vi "PCO_GetExpTrigSignalStatus.vi"(8 "error in (no error)":errorcluster {"code" format="%x"}, 11 "ph":u64) -> (0 "error out":errorcluster {"code" format="%x"}, 1 "wExpTrgSignal":u16(ring) items=["OFF", "ON"], 2 "ErrorMessage":i32 format="%x", 3 "ph out":u64)   [LabVIEW 2019, in "SDK.lvlib" / "TimingControl.lvlib"]
doc: "<b>Description:</b>\nThis function returns the current status of the <exp trig> input line.\nSee respective camera manual for more information about hardware signals.\n\nDue to response and processing times the delay between the software delivered status and the current status may be several milliseconds. For instance caused by interface and / or operating system.\n\n<b>Supported camera type:</b>\npco.pixelfly usb, pco.ultraviolet, pco.1300, pco.1400\n\n<b>Descriptor dependency:</b>\nNone"
uses:
  TimingControl.lvlib
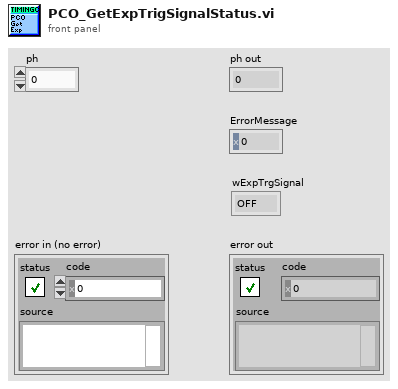
[diagram p1: front panel]
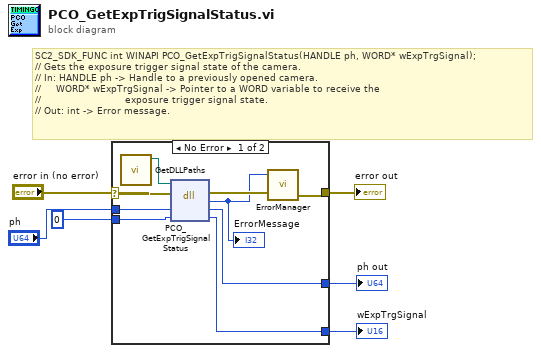
[diagram p0: block diagram]
diagram:
  # "SC2_SDK_FUNC int WINAPI PCO_GetExpTrigSignalStatus(HANDLE ph, WORD* wExpTrgSignal);\n// Gets the exposure trigger signal state of the camera.\n// In: HANDLE ph -> Handle to a previously opened camera.\n//     WORD* wExpTrgSignal -> Pointer to a WORD variable to receive the\n//                            exposure trigger signal state.\n// Out: int -> Error message."
  n1 = case shown="No Error" "error in (no error)" {
    selector: "error in (no error)" -> [w8 w18]
    tunnel: "ph" -> [w15 w17]
    tunnel: [w14 w17] -> w5
    tunnel: u16 0 ("wExpTrgSignal") -> [w13 w16]
    tunnel: [w12 w16] -> w3
    tunnel: [w10 w18] -> w2
    frame No Error {
      n2 = call "GetDLLPaths.vi"() -> ("SC2_Cam_Path"=w7:path)  [unwired: 9 in, 2 out]
      n3 = dll-call lib="?" fn="PCO_GetExpTrigSignalStatus"(path in=w7, error in=w8, "ph"=w15, "wExpTrgSignal"=w13) -> (error out=w11:errorcluster, "return type"=w9:i32, "ph"=w14:u64, "wExpTrgSignal"=w12:u16)  [unwired: 1 in, 1 out]
      "ErrorMessage" <- w9
      n4 = call "ErrorManager.vi"("error in (no error)"=w11, "error code"=w9) -> ("error out"=w10:errorcluster)  [unwired: 3 in]
    }
    frame Error {
    }
  }
  "ph out" <- w5
  "wExpTrgSignal" <- w3
  "error out" <- w2
